vi "Get FPGA for the RUN.vi"(8 "error in (no error)":errorcluster, 10 "index":i32, 11 "Schedule in":refnum<class "Schedule.lvclass">) -> (0 "error out":errorcluster, 2 "FPGA Name":string, 3 "Schedule out":refnum<class "Schedule.lvclass">)   [LabVIEW 2020, in "Run Utilities.lvlib" / "Schedule.lvclass"]
uses:
  Schedule.lvclass
  Schedule.lvclass/Schedule.ctl
  Cell/Schedule Cell.lvclass
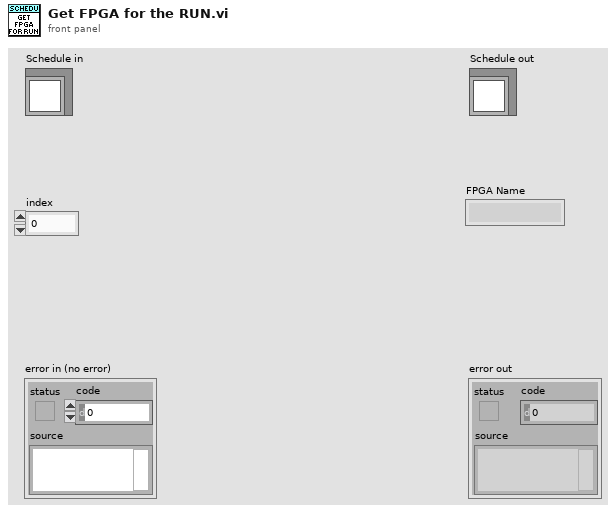
[diagram p1: front panel]
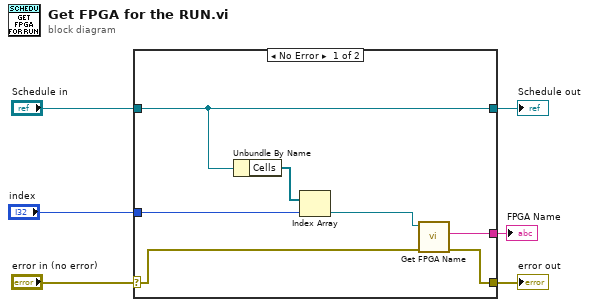
[diagram p0: block diagram]
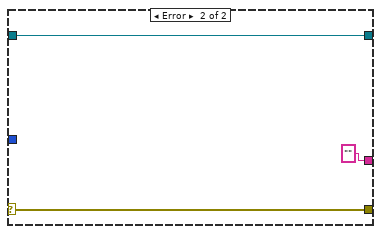
[diagram p2: hidden frame]
diagram:
  n1 = case shown="No Error" "error in (no error)" {
    selector: "error in (no error)" -> [w10 w16]
    tunnel: [w9 w16] -> w5
    tunnel: [w13 w15] -> w3
    tunnel: "Schedule in" -> [w13 w15]
    tunnel: "index" -> [w11 _]
    tunnel: [w8 ""] -> w1
    frame No Error {
      n2 = Unbundle By Name(w13) -> ("Cells"=w12:refnum<class "Schedule Cell.lvclass">[])
      n3 = Index Array(array=w12, index=w11) -> (element=w7:refnum<class "Schedule Cell.lvclass">)
      n4 = call-dynamic "Get FPGA Name.vi"("error in (no error)"=w10, "Schedule Cell in"=w7) -> ("error out"=w9:errorcluster, "FPGA Name"=w8:string)  [unwired: 7 in, 1 out]
    }
    frame Error {
    }
  }
  "error out" <- w5
  "Schedule out" <- w3
  "FPGA Name" <- w1
